vi "Lab13.vi"() -> ()   [LabVIEW 2022 SP3]
uses:
  <vilib>/DAQmx/create/channels.llb/DAQmx Create Channel (CI-Count Edges).vi
  <resource>/objmgr/daqmx.rc
  <vilib>/DAQmx/create/channels.llb/DAQmx Create Channel (CO-Pulse Generation-Frequency).vi
panel:
  in  "stop":bool
  in  "Duty Cycle":dbl=0.5 format="%.6f"
  in  "Input Port":tag
  in  "Output Port":tag
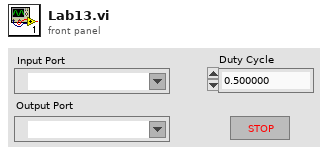
[diagram p1: front panel]
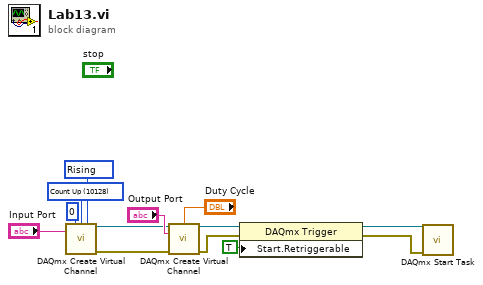
[diagram p0: block diagram]
diagram:
  w12 = 10128 items=["Count Up"=10128, "Count Down"=10124, "Externally Controlled"=10326] ("count direction")
  w13 = 10280 items=["Rising"=10280, "Falling"=10171] ("edge")
  n1 = call-poly <vilib>:"DAQmx Create Virtual Channel.vi"("initial count"=u32 0, "count direction"=w12, "edge"=w13, "counter"="Input Port") -> ("task out"=w6:refnum<k21>, "error out"=w7:errorcluster)  [unwired: 10 in]
  n2 = call-poly <vilib>:"DAQmx Create Virtual Channel.vi"("task in"=w6, "duty cycle"="Duty Cycle", "counter"="Output Port", "error in"=w7) -> ("task out"=w5:refnum<k21>, "error out"=w4:errorcluster)  [unwired: 10 in]
  n3 = property class="DAQmx Trigger"(reference=w5, error in=w4, "Start.Retriggerable"=TRUE) -> (reference out=w3:refnum<k21>, error out=w2:errorcluster)
  n4 = call <vilib>:"DAQmx Start Task.vi"("task/channels in"=w3, "error in"=w2) -> ()  [unwired: 12 in, 2 out]
